vi "Wait StartButton.vi"(8 "error in (no error)":errorcluster) -> (0 "error out":errorcluster)   [LabVIEW 2024]
uses:
  Ctrl/PLC Enum.ctl
panel:
  out "Status?":bool
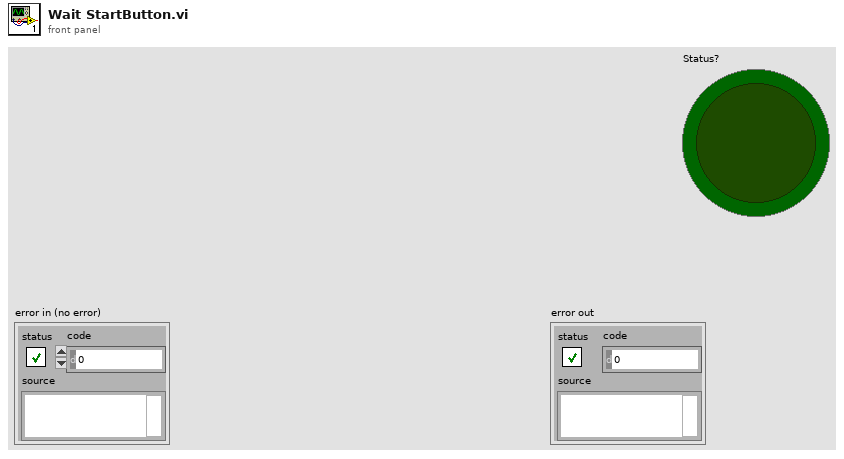
[diagram p1: front panel]
types:
  T1 = typedef "PLC Enum.ctl" = enum16{"Init", "Enable", "Orign", "Load", "Start", "Stop", "StartTest", "StopTest", "Reflector", "WriteResult", "SetSpeed", "SetOrign", "SetLoad", "ServoStatus?", "EquipStatus?", "Origin?", "TestStatus?", "Loadstatus?", "DUTStatus?", "Mes?", "Error？", "Position？", "Speed?", "PinCount", "RunMode", "SN", "Reset", "Jog+", "Jog-", "Close", "Up", "Down", "Clamp", "Release", "In", "Out", "EnterTestMode", "ExitTestMode", "StartButton", "ScanOK", "Power"}
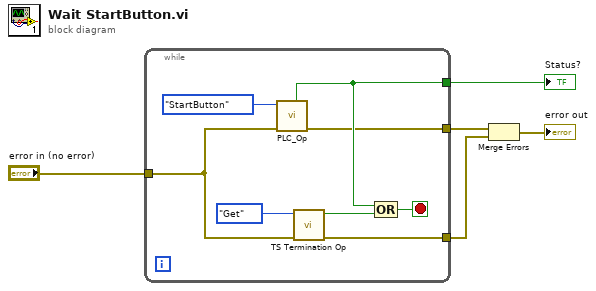
[diagram p0: block diagram]
diagram:
  n1 = while {
    tunnel: [w9] -> w5
    tunnel: "error in (no error)" -> [w8]
    tunnel: [w12] -> w4
    tunnel: [w7] -> w3
    stop <- w13 stop-if-true
    n2 = call "PLC_Op.vi"("error in (no error)"=w8, "Status"=PLC_Enum."StartButton") -> ("error out"=w7:errorcluster, "Boolean 2"=w9:bool)  [unwired: 4 in, 4 out]
    n3 = call "TS Termination Op.vi"("error in (no error)"=w8, "Enum"=enum16{"Initialize", "Get", "Close"}."Get") -> ("error out"=w12:errorcluster, "Terminating or Aborting"=w11:bool)  [unwired: 8 in]
    n4 = Compound Arithmetic op=OR(w9, w11) -> (w13:bool)
  }
  "Status?" <- w5
  n5 = Merge Errors(w3, w4) -> (→"error out":errorcluster)
